vi "Shoot Joystick.vi"(11 "Operator Right Trigger":dbl) -> (3 "Shoot Teleop Command":T1)   [LabVIEW 2019]
uses:
  Shoot/Shooter Mode Type Def.ctl
  Shoot/Shooter Command Type Def.ctl
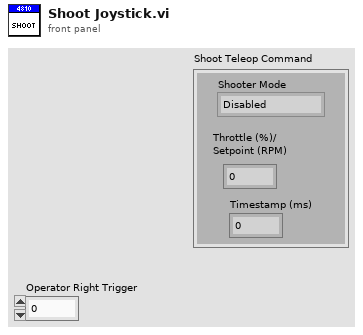
[diagram p1: front panel]
types:
  T1 = typedef "Shooter Command Type Def.ctl" = cluster{"Shooter Mode":T2, "Throttle (%)/ \nSetpoint (RPM)":dbl, "Timestamp (ms)":dbl}
  T2 = typedef "Shooter Mode Type Def.ctl" = enum16{"Disabled", "Raw Throttle", "Velocity Control"}
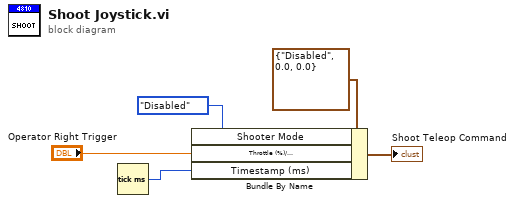
[diagram p0: block diagram]
diagram:
  n1 = Tick Count (ms)() -> (millisecond timer value=w1:u32)
  n2 = Bundle By Name(cluster=T1 {"Shooter Mode"=enum."Disabled", "Throttle (%)/ \nSetpoint (RPM)"=0.0, "Timestamp (ms)"=0.0} ("Teleop Shooter Command"), "Shooter Mode"=Shooter_Mode_Type_Def."Disabled", "Throttle (%)/ \nSetpoint (RPM)"="Operator Right Trigger", "Timestamp (ms)"=w1) -> (→"Shoot Teleop Command":T1)
